vi "Arm Actuator Controller.vi"(8 "error in":errorcluster) -> ()   [LabVIEW 2017]
doc: "This VI executes continuously carrying out the current operation and responding to updates or new operations. It will often contain the timing or control code that is difficult to place directly in TeleOp. This VI generally opens all sensors and motors and isolates the rest of the robot code from knowing how the operations are carried out."
uses:
  Arm Actuator Setpoints.ctl
  Arm Actuator Operations.ctl
  Public/Documents/Cross The Road Electronics/Phoenix-LabVIEW/Motor Controller/Controls/CTRE_Phoenix_MotorControl_ControlMode.ctl
  <vilib>/Rock Robotics/WPI/ThirdParty/Phoenix-LabVIEW/Motor Controller/Controls/CTRE_Phoenix_MotorControl_NeutralMode.ctl
  <vilib>/Rock Robotics/WPI/Solenoid/WPI_SolenoidValue.ctl
  <vilib>/Rock Robotics/WPI/Solenoid/WPI_SolenoidChannel.ctl
  <vilib>/Rock Robotics/WPI/Solenoid/WPI_SolenoidOpenSingle.vi
  <vilib>/Rock Robotics/WPI/Solenoid/WPI_SolenoidSetEnum.vi
  <vilib>/Rock Robotics/Network Tables/NT Read Number.vi
  <vilib>/addons/control/pid/pid.llb/PID (DBL).vi
  <vilib>/addons/control/pid/NI_PID_pid.lvlib
  <vilib>/Rock Robotics/Network Tables/NT Write Boolean.vi
panel:
  out "Current\nCmd":string
  # "Tip: It may be helpful to observe inputs and sensor values.\nYou may also want to display tuning or debugging controls."
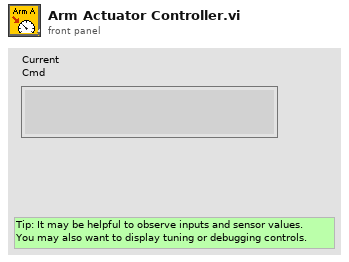
[diagram p1: front panel]
types:
  T1 = typedef "WPI_SolenoidChannel.ctl" = enum8{"Solenoid 0", "Solenoid 1", "Solenoid 2", "Solenoid 3", "Solenoid 4", "Solenoid 5", "Solenoid 6", "Solenoid 7", "Invalid"}
  T2 = typedef "WPI_SolenoidValue.ctl" = enum16{"Off", "On", "Forward", "Reverse"}
  T3 = typedef "CTRE_Phoenix_MotorControl_NeutralMode.ctl" = enum8{"EEPROMSetting", "Override to Coast", "Override to Brake"}
  T4 = typedef "CTRE_Phoenix_MotorControl_ControlMode.ctl" = u16
  T5 = typedef "Arm Actuator Setpoints.ctl" = cluster{"Operation":T6, "Setpoint":dbl, "Duration":dbl, "POT":dbl, "Arm Out Allowed?":bool}
  T6 = typedef "Arm Actuator Operations.ctl" = enum16{"Reserve", "Read Current", "Immediate", "Move Arm", "Claw In", "Claw Out", "Preset"}
  T7 = typedef "WPI_MotorControlDeviceRef.ctl" = cluster{"DeviceStatus":errorcluster, "Type":T8, "PWM":cluster{"PWM Channel":T9, "DeadBand":T10}, "CAN":cluster{"Device Number":u8, "SetOutput VI Ref":variant, "GetOutput VI Ref":variant, "Enable VI Ref":variant, "Disable VI Ref":variant, "Data":variant}, "Invert":bool, "DIO PWM":cluster{"PWM \"Enable\" Channel":T9, "DIOChannel":T11, "PWM Rate":dbl}}
  T8 = typedef "WPI_MotorControlType.ctl" = enum16{"PWM", "CAN", "DIO PWM"}
  T9 = typedef "FPGA_DIOPWMChannel.ctl" = enum8{"PWM 0", "PWM 1", "PWM 2", "PWM 3", "PWM 4", "PWM 5", "PWM 6", "PWM 7", "PWM 8", "PWM 9", "PWM MXP 0", "PWM MXP 1", "PWM MXP 2", "PWM MXP 3", "PWM MXP 4", "PWM MXP 5", "PWM MXP 6", "PWM MXP 7", "PWM MXP 8", "PWM MXP 9", "Invalid"}
  T10 = typedef "WPI_PWMDeadband.ctl" = cluster{"Name":string, "maxPositivePwm":i32, "minPositivePwm":i32, "centerPwm":i32, "maxNegativePwm":i32, "minNegativePwm":i32, "angularRange":u16}
  T11 = typedef "FPGA_DIOChannel.ctl" = enum8{"DIO 0", "DIO 1", "DIO 2", "DIO 3", "DIO 4", "DIO 5", "DIO 6", "DIO 7", "DIO 8", "DIO 9", "DIO MXP 0", "DIO MXP 1", "DIO MXP 2", "DIO MXP 3", "DIO MXP 4", "DIO MXP 5", "DIO MXP 6", "DIO MXP 7", "DIO MXP 8", "DIO MXP 9", "DIO MXP 10", "DIO MXP 11", "DIO MXP 12", "DIO MXP 13", "DIO MXP 14", "DIO MXP 15", "SPI Port CS1", "SPI Port CS2", "SPI Port CS3", "SPI Port MISO", "SPI Port MOSI", "Invalid"}
  T12 = typedef "WPI_SolenoidDevRef.ctl" = cluster{"DevStatus":errorcluster, "Pneumatics Control Module":u8, "Forward Solenoid Channel":T1, "Reverse Solenoid Channel":T1}
  T13 = typedef "Command Status Info.ctl" = cluster{"Name":string, "Status":T14, "notifier out":T15}
  T14 = typedef "Completion Status.ctl" = enum16{"Successful", "Aborted", "Incomplete"}
  T15 = typedef "Completion Notifier.ctl" = refnum<notifier>
  T16 = cluster{"Current Command":T5, "Command Timing":cluster{"Start Time (ms)":u32, "Iterations":i32}, "Command Arguments":cluster{"Command Info":T13, "Description":string, "Default Command":T5, "queue out":refnum<queue>, "Subsystem Name":string}}
  T17 = enum16{"FollowerType_PercentOutput", "FollowerType_AuxOutput1"}
  T18 = cluster{"proportional gain (Kc)":dbl, "integral time (Ti, min)":dbl, "derivative time (Td, min)":dbl}
  T19 = typedef "WPI_AnalogChannelDevRef.ctl" = cluster{"DevStatus":errorcluster, "Analog Channel":T20}
  T20 = typedef "FPGA_AIChannel.ctl" = enum8{"AI 0", "AI 1", "AI 2", "AI 3", "AI MXP 0", "AI MXP 1", "AI MXP 2", "AI MXP 3", "Invalid"}
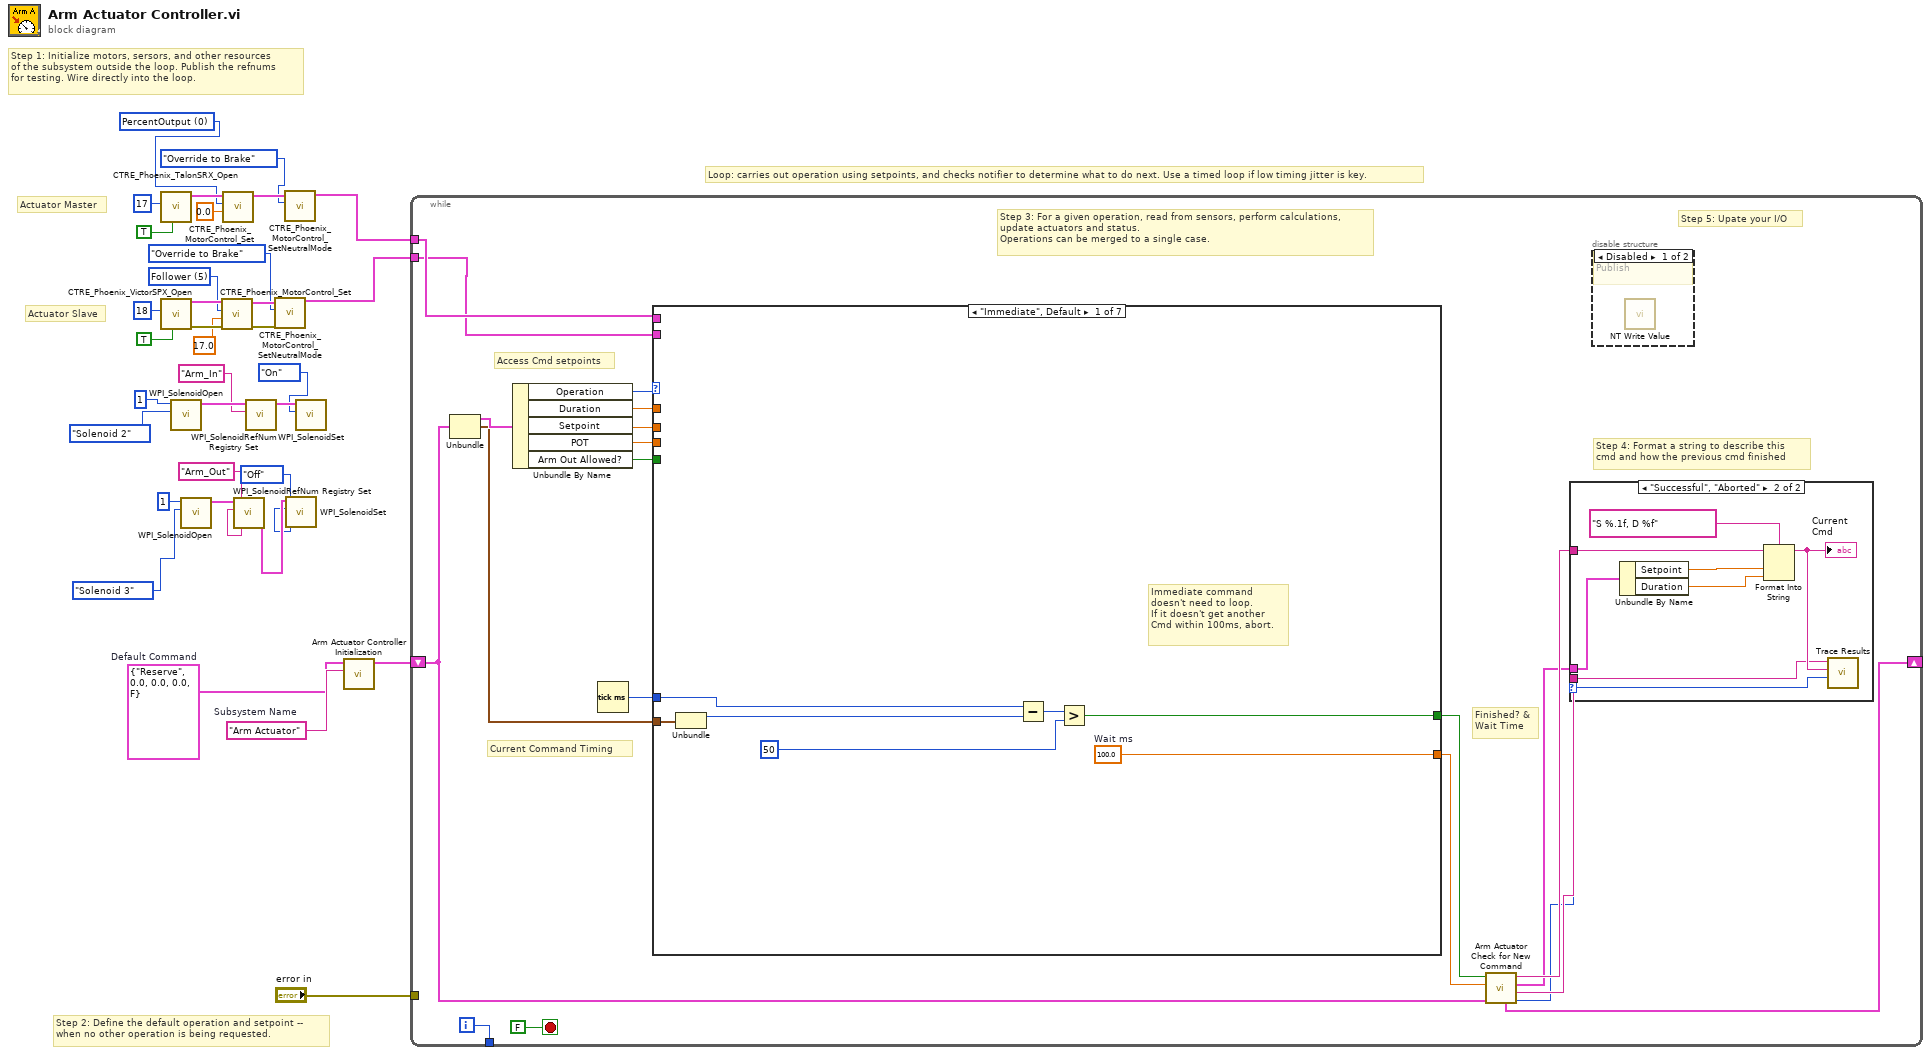
[diagram p0: block diagram]
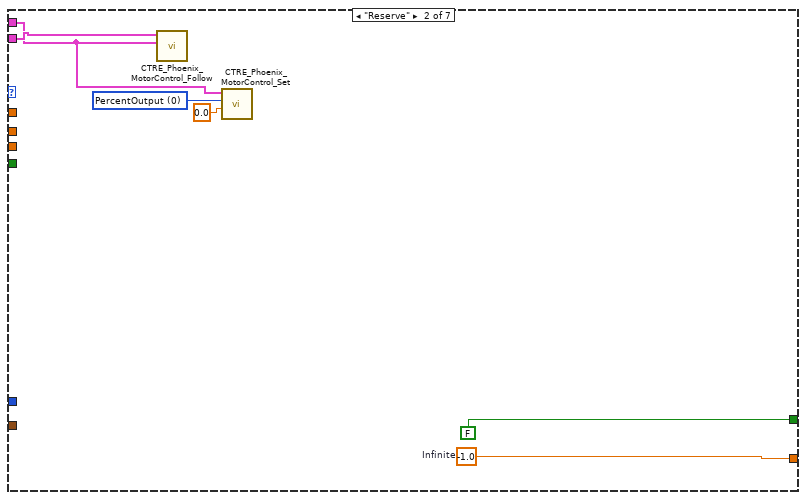
[diagram p4: hidden frame]
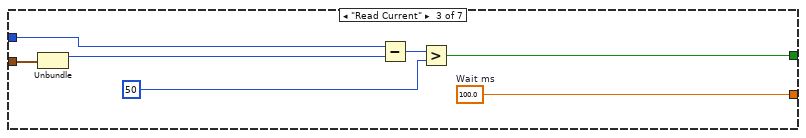
[diagram p5: hidden frame]
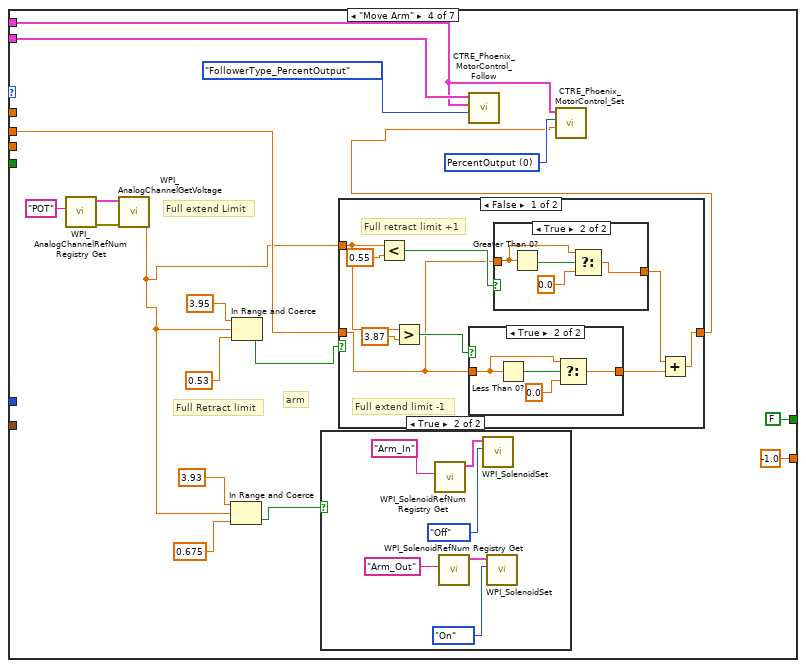
[diagram p6: hidden frame]
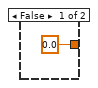
[diagram p8: hidden frame]
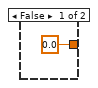
[diagram p9: hidden frame]
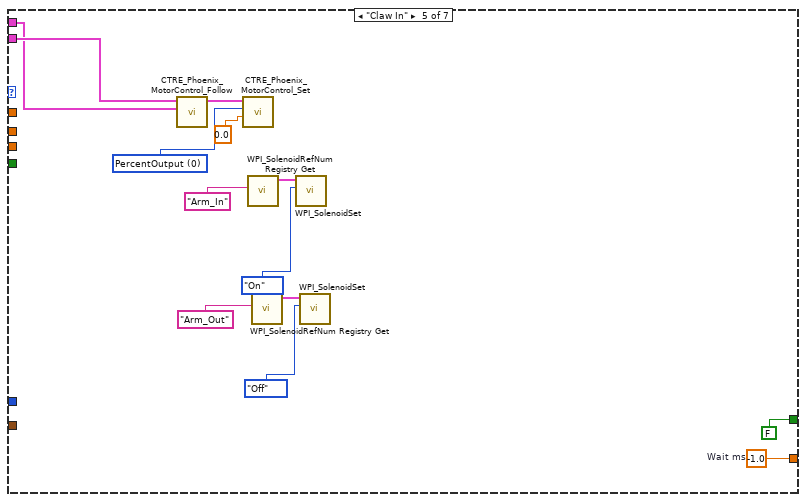
[diagram p11: hidden frame]
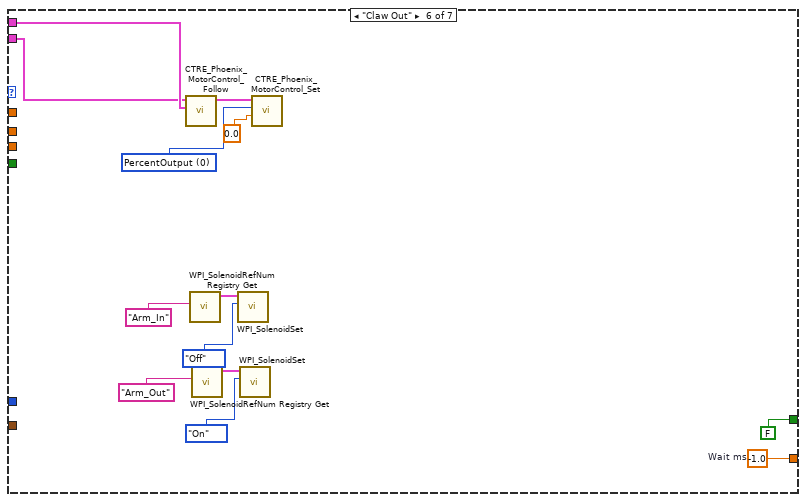
[diagram p12: hidden frame]
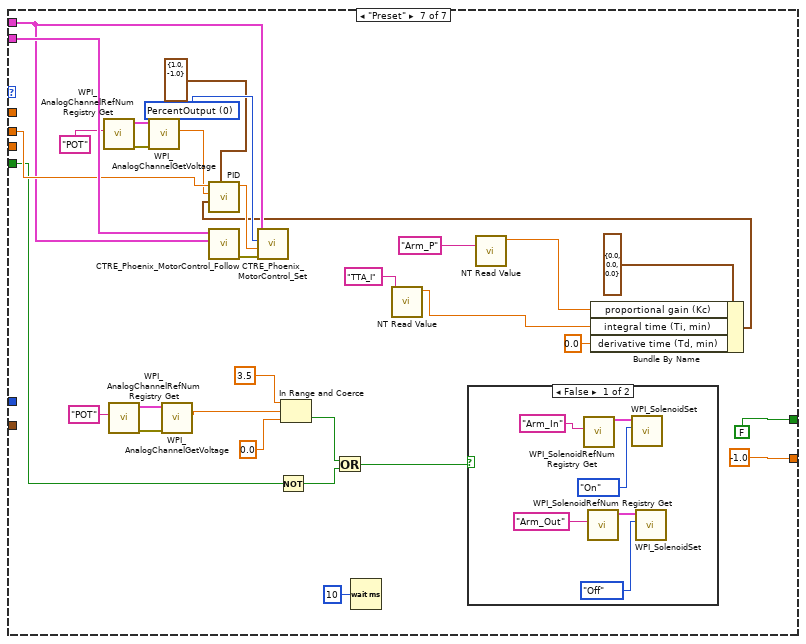
[diagram p13: hidden frame]
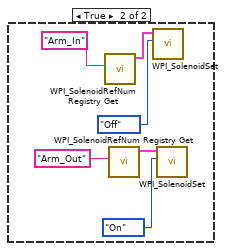
[diagram p14: hidden frame]
diagram:
  w16 = T4 5 items=["PercentOutput"=0, "Position"=1, "Velocity"=2, "Current"=3, "Follower"=5, "MotionProfile"=6, "MotionMagic"=7, "MotionMagicArc"=8, "MotionProfileArc"=10, "Disabled"=15] ("Control Mode")
  w23 = T4 0 items=["PercentOutput"=0, "Position"=1, "Velocity"=2, "Current"=3, "Follower"=5, "MotionProfile"=6, "MotionMagic"=7, "MotionMagicArc"=8, "MotionProfileArc"=10, "Disabled"=15] ("Control Mode")
  w31 = T5 {"Operation"=enum."Reserve", "Setpoint"=0.0, "Duration"=0.0, "POT"=0.0, "Arm Out Allowed?"=FALSE}  # Default Command
  w32 = "Arm Actuator"  # Subsystem Name
  # "Actuator Slave"
  # "Actuator Master"
  # "Step 2: Define the default operation and setpoint --\nwhen no other operation is being requested."
  # "Step 1: Initialize motors, sersors, and other resources\nof the subsystem outside the loop. Publish the refnums\nfor testing. Wire directly into the loop."
  # "Loop: carries out operation using setpoints, and checks notifier to determine what to do next. Use a timed loop if low timing jitter is key."
  n1 = call <vilib>:"CTRE_Phoenix_TalonSRX_Open.vi"("Invert"=TRUE, "Device Number"=u8 17) -> ("CAN Talon SRX Ref"=w24:T7)  [unwired: 8 in, 1 out]
  n2 = call <vilib>:"CTRE_Phoenix_VictorSPX_Open.vi"("Invert"=TRUE, "Device Number"=u8 18) -> ("error out"=w18:errorcluster, "CAN Talon SRX Ref"=w17:T7)  [unwired: 8 in]
  n3 = call-poly <vilib>:"WPI_SolenoidOpen.vi"("Solenoid Channel"=WPI_SolenoidChannel."Solenoid 2", "Pneumatics Control Module (0)"=u8 1) -> ("SolenoidDevRef"=w30:T12)  [unwired: 8 in, 1 out]
  n4 = call-poly <vilib>:"WPI_SolenoidOpen.vi"("Solenoid Channel"=WPI_SolenoidChannel."Solenoid 3", "Pneumatics Control Module (0)"=u8 1) -> ("SolenoidDevRef"=w28:T12)  [unwired: 8 in, 1 out]
  n5 = call <vilib>:"CTRE_Phoenix_MotorControl_Set.vi"("error in (no error)"=w18, "Output"=17.0, "Control Mode"=w16, "PhoenixMotorControlDevRef"=w17) -> ("error out"=w14:errorcluster, "PhoenixMotorControlDevRef"=w13:T7)  [unwired: 6 in]
  n6 = call <vilib>:"CTRE_Phoenix_MotorControl_Set.vi"("Output"=0.0, "Control Mode"=w23, "PhoenixMotorControlDevRef"=w24) -> ("PhoenixMotorControlDevRef"=w21:T7)  [unwired: 7 in, 1 out]
  n7 = call <vilib>:"WPI_SolenoidRefNum Registry Set.vi"("refnum name"="Arm_Out", "SolenoidDevRef"=w28) -> ("SolenoidDevRef"=w9:T12)  [unwired: 8 in, 1 out]
  n8 = call <vilib>:"WPI_SolenoidRefNum Registry Set.vi"("refnum name"="Arm_In", "SolenoidDevRef"=w30) -> ("SolenoidDevRef"=w7:T12)  [unwired: 8 in, 1 out]
  n9 = call <vilib>:"CTRE_Phoenix_MotorControl_SetNeutralMode.vi"("error in (no error)"=w14, "Motor Control Neutral Mode"=CTRE_Phoenix_MotorControl_NeutralMode."Override to Brake", "PhoenixMotorControlDevRef"=w13) -> ("PhoenixMotorControlDevRef"=w10:T7)  [unwired: 7 in, 1 out]
  n10 = call <vilib>:"CTRE_Phoenix_MotorControl_SetNeutralMode.vi"("Motor Control Neutral Mode"=CTRE_Phoenix_MotorControl_NeutralMode."Override to Brake", "PhoenixMotorControlDevRef"=w21) -> ("PhoenixMotorControlDevRef"=w11:T7)  [unwired: 8 in, 1 out]
  n11 = call-poly <vilib>:"WPI_SolenoidSet.vi"("Value"=WPI_SolenoidValue."Off", "SolenoidDevRef"=w9) -> ()  [unwired: 8 in, 2 out]
  n12 = call-poly <vilib>:"WPI_SolenoidSet.vi"("Value"=WPI_SolenoidValue."On", "SolenoidDevRef"=w7) -> ()  [unwired: 8 in, 2 out]
  n13 = call "Arm Actuator Controller Initialization.vi"("Subsystem Name"=w32, "Default Command"=w31) -> ("Current Command"=w33:T16)  [unwired: 9 in]
  n14 = while {
    shift-right: [w46] -> _
    shift-left: w33 -> [w39]
    tunnel: [w53] -> _
    tunnel: "error in" -> [_]
    tunnel: w11 -> [w38]
    tunnel: w10 -> [w37]
    i -> [w53]
    stop <- FALSE stop-if-true
    # "Step 5: Upate your I/O"
    # "Step 4: Format a string to describe this\ncmd and how the previous cmd finished"
    # "Current Command Timing"
    # "Access Cmd setpoints"
    # "Finished? &\nWait Time"
    # "Step 3: For a given operation, read from sensors, perform calculations,\nupdate actuators and status.\nOperations can be merged to a single case."
    n15 = Unbundle(w39) -> ("Current Command"=w52:T5, "Command Timing"=w48:cluster{"Start Time (ms)":u32, "Iterations":i32})  [unwired: 1 out]
    n16 = Unbundle By Name(w52) -> ("Operation"=w51:T6, "Duration"=w50:dbl, "Setpoint"=w47:dbl, "POT"=w36:dbl, "Arm Out Allowed?"=w35:bool)
    n17 = Tick Count (ms)() -> (millisecond timer value=w49:u32)
    n18 = case shown="\"Immediate\", Default" w51 {
      tunnel: [w69 w75 w77 -1.0 ("Wait ms") w139 w152 -1.0 ("Wait ms")] -> w44
      tunnel: [w63 FALSE ("ignore previous (F)") w78 FALSE ("ignore previous (F)") FALSE ("ignore previous (F)") FALSE ("ignore previous (F)") FALSE ("ignore previous (F)")] -> w45
      tunnel: w48 -> [w65 _ w76 _ _ _ _]
      tunnel: w50 -> [_ _ _ _ _ _ _]
      tunnel: w49 -> [w64 _ w79 _ _ _ _]
      tunnel: w47 -> [_ _ _ w91 _ _ w179]
      tunnel: w38 -> [_ w70 _ w96 w134 w148 w177]
      tunnel: w37 -> [_ w73 _ w99 w135 w147 w180]
      tunnel: w36 -> [_ _ _ _ _ _ _]
      tunnel: w35 -> [_ _ _ _ _ _ w161]
      frame "Immediate", Default {
        w69 = 100.0  # Wait ms
        # "Immediate command\ndoesn't need to loop.\nIf it doesn't get another\nCmd within 100ms, abort."
        n19 = Unbundle(w65) -> ("Start Time (ms)"=w68:u32)  [unwired: 1 out]
        n20 = Subtract(x=w64, y=w68) -> (x-y=w67:u32)
        n21 = Greater?(x=w67, y=u8 50 ("Left Motor")) -> (0:w63:bool)
      }
      frame "Reserve" {
        w71 = T4 0 items=["PercentOutput"=0, "Position"=1, "Velocity"=2, "Current"=3, "Follower"=5, "MotionProfile"=6, "MotionMagic"=7, "MotionMagicArc"=8, "MotionProfileArc"=10, "Disabled"=15] ("Control Mode")
        w75 = -1.0  # Infinite
        n22 = call <vilib>:"CTRE_Phoenix_MotorControl_Follow.vi"("Master Controller to Follow"=w70, "PhoenixMotorControlDevRef"=w73) -> ()  [unwired: 8 in, 2 out]
        n23 = call <vilib>:"CTRE_Phoenix_MotorControl_Set.vi"("Output"=0.0, "Control Mode"=w71, "PhoenixMotorControlDevRef"=w70) -> ()  [unwired: 7 in, 2 out]
      }
      frame "Read Current" {
        w77 = 100.0  # Wait ms
        n24 = Unbundle(w76) -> ("Start Time (ms)"=w82:u32)  [unwired: 1 out]
        n25 = Subtract(x=w79, y=w82) -> (x-y=w81:u32)
        n26 = Greater?(x=w81, y=u8 50 ("Left Motor")) -> (0:w78:bool)
      }
      frame "Move Arm" {
        w100 = T4 0 items=["PercentOutput"=0, "Position"=1, "Velocity"=2, "Current"=3, "Follower"=5, "MotionProfile"=6, "MotionMagic"=7, "MotionMagicArc"=8, "MotionProfileArc"=10, "Disabled"=15] ("Control Mode")
        # "arm"
        # "Full Retract limit"
        # "Full extend Limit"
        n27 = call <vilib>:"WPI_AnalogChannelRefNum Registry Get.vi"("refnum name"="POT") -> ("error out"=w95:errorcluster, "AIDeviceRef"=w94:T19)  [unwired: 9 in]
        n28 = call <vilib>:"WPI_AnalogChannelGetVoltage.vi"("error in (no error)"=w95, "AIDeviceRef"=w94) -> ("Voltage"=w88:dbl)  [unwired: 7 in, 2 out]
        n29 = In Range and Coerce(upper limit=3.93 ("y"), x=w88, lower limit=0.675) -> (In Range?=w89:bool)  [unwired: 1 out]
        n30 = In Range and Coerce(upper limit=3.95, x=w88, lower limit=0.53) -> (In Range?=w92:bool)  [unwired: 1 out]
        n31 = case shown="True" w89 {
          frame False {
          }
          frame True {
            n32 = call <vilib>:"WPI_SolenoidRefNum Registry Get.vi"("refnum name"="Arm_In") -> ("SolenoidDevRef"=w101:T12)  [unwired: 9 in, 1 out]
            n33 = call <vilib>:"WPI_SolenoidRefNum Registry Get.vi"("refnum name"="Arm_Out") -> ("SolenoidDevRef"=w102:T12)  [unwired: 9 in, 1 out]
            n34 = call-poly <vilib>:"WPI_SolenoidSet.vi"("Value"=WPI_SolenoidValue."Off", "SolenoidDevRef"=w101) -> ()  [unwired: 8 in, 2 out]
            n35 = call-poly <vilib>:"WPI_SolenoidSet.vi"("Value"=WPI_SolenoidValue."On", "SolenoidDevRef"=w102) -> ()  [unwired: 8 in, 2 out]
          }
        }
        n36 = case shown="False" w92 {
          tunnel: w91 -> [w107 w126]
          tunnel: [w111 w126] -> w87
          tunnel: w88 -> [w108 _]
          frame False {
            # "Full extend limit -1"
            # "Full retract limit +1"
            n37 = Less?(x=w108, y=0.55) -> (x < y?=w109:bool)
            n38 = Greater?(x=w108, y=3.87) -> (0:w110:bool)
            n39 = case shown="True" w110 {
              tunnel: [0.0 ("f") w120] -> w113
              tunnel: w107 -> [_ w118]
              frame False {
              }
              frame True {
                n40 = Less Than 0?(x=w118) -> (x < 0?=w119:bool)
                n41 = Select(t=w118, s=w119, f=0.0) -> (s? t:f=w120:dbl)
              }
            }
            n42 = case shown="True" w109 {
              tunnel: [0.0 ("f") w124] -> w114
              tunnel: w107 -> [_ w123]
              frame False {
              }
              frame True {
                n43 = Greater Than 0?(x=w123) -> (x > 0?=w125:bool)
                n44 = Select(t=w123, s=w125, f=0.0) -> (s? t:f=w124:dbl)
              }
            }
            n45 = Add(x=w114, y=w113) -> (x+y=w111:dbl)
          }
          frame True {
          }
        }
        n46 = call <vilib>:"CTRE_Phoenix_MotorControl_Follow.vi"("FollowerType"=T17."FollowerType_PercentOutput", "Master Controller to Follow"=w96, "PhoenixMotorControlDevRef"=w99) -> ()  [unwired: 7 in, 2 out]
        n47 = call <vilib>:"CTRE_Phoenix_MotorControl_Set.vi"("Output"=w87, "Control Mode"=w100, "PhoenixMotorControlDevRef"=w96) -> ()  [unwired: 7 in, 2 out]
      }
      frame "Claw In" {
        w136 = T4 0 items=["PercentOutput"=0, "Position"=1, "Velocity"=2, "Current"=3, "Follower"=5, "MotionProfile"=6, "MotionMagic"=7, "MotionMagicArc"=8, "MotionProfileArc"=10, "Disabled"=15] ("Control Mode")
        w139 = -1.0  # Wait ms
        n48 = call <vilib>:"CTRE_Phoenix_MotorControl_Follow.vi"("Master Controller to Follow"=w134, "PhoenixMotorControlDevRef"=w135) -> ("PhoenixMotorControlDevRef"=w138:T7)  [unwired: 8 in, 1 out]
        n49 = call <vilib>:"CTRE_Phoenix_MotorControl_Set.vi"("Output"=0.0, "Control Mode"=w136, "PhoenixMotorControlDevRef"=w138) -> ()  [unwired: 7 in, 2 out]
        n50 = call <vilib>:"WPI_SolenoidRefNum Registry Get.vi"("refnum name"="Arm_In") -> ("SolenoidDevRef"=w130:T12)  [unwired: 9 in, 1 out]
        n51 = call <vilib>:"WPI_SolenoidRefNum Registry Get.vi"("refnum name"="Arm_Out") -> ("SolenoidDevRef"=w128:T12)  [unwired: 9 in, 1 out]
        n52 = call-poly <vilib>:"WPI_SolenoidSet.vi"("Value"=WPI_SolenoidValue."On", "SolenoidDevRef"=w130) -> ()  [unwired: 8 in, 2 out]
        n53 = call-poly <vilib>:"WPI_SolenoidSet.vi"("Value"=WPI_SolenoidValue."Off", "SolenoidDevRef"=w128) -> ()  [unwired: 8 in, 2 out]
      }
      frame "Claw Out" {
        w149 = T4 0 items=["PercentOutput"=0, "Position"=1, "Velocity"=2, "Current"=3, "Follower"=5, "MotionProfile"=6, "MotionMagic"=7, "MotionMagicArc"=8, "MotionProfileArc"=10, "Disabled"=15] ("Control Mode")
        w152 = -1.0  # Wait ms
        n54 = call <vilib>:"CTRE_Phoenix_MotorControl_Follow.vi"("Master Controller to Follow"=w148, "PhoenixMotorControlDevRef"=w147) -> ("PhoenixMotorControlDevRef"=w151:T7)  [unwired: 8 in, 1 out]
        n55 = call <vilib>:"WPI_SolenoidRefNum Registry Get.vi"("refnum name"="Arm_In") -> ("SolenoidDevRef"=w142:T12)  [unwired: 9 in, 1 out]
        n56 = call <vilib>:"WPI_SolenoidRefNum Registry Get.vi"("refnum name"="Arm_Out") -> ("SolenoidDevRef"=w140:T12)  [unwired: 9 in, 1 out]
        n57 = call-poly <vilib>:"WPI_SolenoidSet.vi"("Value"=WPI_SolenoidValue."Off", "SolenoidDevRef"=w142) -> ()  [unwired: 8 in, 2 out]
        n58 = call-poly <vilib>:"WPI_SolenoidSet.vi"("Value"=WPI_SolenoidValue."On", "SolenoidDevRef"=w140) -> ()  [unwired: 8 in, 2 out]
        n59 = call <vilib>:"CTRE_Phoenix_MotorControl_Set.vi"("Output"=0.0, "Control Mode"=w149, "PhoenixMotorControlDevRef"=w151) -> ()  [unwired: 7 in, 2 out]
      }
      frame "Preset" {
        w181 = T4 0 items=["PercentOutput"=0, "Position"=1, "Velocity"=2, "Current"=3, "Follower"=5, "MotionProfile"=6, "MotionMagic"=7, "MotionMagicArc"=8, "MotionProfileArc"=10, "Disabled"=15] ("Control Mode")
        n60 = call <vilib>:"WPI_AnalogChannelRefNum Registry Get.vi"("refnum name"="POT") -> ("error out"=w175:errorcluster, "AIDeviceRef"=w174:T19)  [unwired: 9 in]
        n61 = call <vilib>:"WPI_AnalogChannelRefNum Registry Get.vi"("refnum name"="POT") -> ("error out"=w170:errorcluster, "AIDeviceRef"=w169:T19)  [unwired: 9 in]
        n62 = call <vilib>:"WPI_AnalogChannelGetVoltage.vi"("error in (no error)"=w175, "AIDeviceRef"=w174) -> ("Voltage"=w172:dbl)  [unwired: 7 in, 2 out]
        n63 = call <vilib>:"WPI_AnalogChannelGetVoltage.vi"("error in (no error)"=w170, "AIDeviceRef"=w169) -> ("Voltage"=w165:dbl)  [unwired: 7 in, 2 out]
        n64 = call <vilib>:"CTRE_Phoenix_MotorControl_Follow.vi"("Master Controller to Follow"=w177, "PhoenixMotorControlDevRef"=w180) -> ("error out"=w176:errorcluster)  [unwired: 8 in, 1 out]
        n65 = Not(x=w161) -> (.not. x?=w162:bool)
        n66 = In Range and Coerce(upper limit=3.5 ("y"), x=w165, lower limit=0.0) -> (In Range?=w164:bool)  [unwired: 1 out]
        n67 = Or(x=w164, y=w162) -> (x .or. y?=w163:bool)
        n68 = Wait (ms)(milliseconds to wait=u32 10) -> ()  [unwired: 1 out]
        n69 = call-poly <vilib>:"NT Read Value.vi"("Name"="TTA_I") -> ("Numeric"=w158:dbl)  [unwired: 9 in, 1 out]
        n70 = case shown="False" w163 {
          frame False {
            n71 = call <vilib>:"WPI_SolenoidRefNum Registry Get.vi"("refnum name"="Arm_In") -> ("SolenoidDevRef"=w185:T12)  [unwired: 9 in, 1 out]
            n72 = call <vilib>:"WPI_SolenoidRefNum Registry Get.vi"("refnum name"="Arm_Out") -> ("SolenoidDevRef"=w189:T12)  [unwired: 9 in, 1 out]
            n73 = call-poly <vilib>:"WPI_SolenoidSet.vi"("Value"=WPI_SolenoidValue."On", "SolenoidDevRef"=w185) -> ()  [unwired: 8 in, 2 out]
            n74 = call-poly <vilib>:"WPI_SolenoidSet.vi"("Value"=WPI_SolenoidValue."Off", "SolenoidDevRef"=w189) -> ()  [unwired: 8 in, 2 out]
          }
          frame True {
            n75 = call <vilib>:"WPI_SolenoidRefNum Registry Get.vi"("refnum name"="Arm_In") -> ("SolenoidDevRef"=w190:T12)  [unwired: 9 in, 1 out]
            n76 = call <vilib>:"WPI_SolenoidRefNum Registry Get.vi"("refnum name"="Arm_Out") -> ("SolenoidDevRef"=w191:T12)  [unwired: 9 in, 1 out]
            n77 = call-poly <vilib>:"WPI_SolenoidSet.vi"("Value"=WPI_SolenoidValue."Off", "SolenoidDevRef"=w190) -> ()  [unwired: 8 in, 2 out]
            n78 = call-poly <vilib>:"WPI_SolenoidSet.vi"("Value"=WPI_SolenoidValue."On", "SolenoidDevRef"=w191) -> ()  [unwired: 8 in, 2 out]
          }
        }
        n79 = call-poly <vilib>:"NT Read Value.vi"("Name"="Arm_P") -> ("Numeric"=w159:dbl)  [unwired: 9 in, 1 out]
        n80 = Bundle By Name(cluster=T18 {"proportional gain (Kc)"=0.0, "integral time (Ti, min)"=0.0, "derivative time (Td, min)"=0.0} ("PID gains"), "proportional gain (Kc)"=w159, "integral time (Ti, min)"=w158, "derivative time (Td, min)"=0.0) -> (w155:T18)
        n81 = call-poly <vilib>:"PID.vi"("output range"=cluster{"output high":dbl, "output low":dbl} {"output high"=1.0, "output low"=-1.0}, "PID gains"=w155, "process variable"=w172, "setpoint"=w179) -> ("output"=w178:dbl)  [unwired: 6 in, 1 out]
        n82 = call <vilib>:"CTRE_Phoenix_MotorControl_Set.vi"("error in (no error)"=w176, "Output"=w178, "Control Mode"=w181, "PhoenixMotorControlDevRef"=w177) -> ()  [unwired: 6 in, 2 out]
      }
    }
    n83 = call "Arm Actuator Check for New Command.vi"("Current Command"=w39, "Wait time (ms)"=w44, "Finished?"=w45) -> ("Completion"=w40:T14, "Subsystem Name"=w41:string, "Current Command"=w42:T5, "Initial Trace String"=w43:string, "NextCommand"=w46:T16)  [unwired: 4 in]
    n84 = case shown="\"Successful\", \"Aborted\"" w40 {
      selector: w40 -> [_ w62]
      tunnel: w43 -> [_ w58]
      tunnel: w42 -> [_ w59]
      tunnel: w41 -> [_ w55]
      frame "Incomplete", Default {
        # "Continuing current command"
      }
      frame "Successful", "Aborted" {
        # "Report and setup for next command"
        n85 = Unbundle By Name(w59) -> ("Setpoint"=w61:dbl, "Duration"=w56:dbl)
        n86 = Format Into String(format string="S %.1f, D %f", initial string=w58, w61, w56) -> (resulting string=w57:string)  [unwired: 1 in, 1 out]
        "Current\nCmd" <- w57
        n87 = call <vilib>:"Trace Results.vi"("Status of previous command"=w62, "Description"=w57, "Subsystem"=w55) -> ()  [unwired: 9 in]
      }
    }
    n88 = disable-structure shown="Disabled" {
      frame Disabled {
        # "Publish"
        n89 = call-poly <vilib>:"NT Write Value.vi"() -> ()  [unwired: 11 in, 1 out]
      }
      frame Enabled {
      }
    }
  }
